vi "Query Multi Eval Meas List Power Spectral Density Limit Check Results.vi"(8 "error in (no error)":errorcluster, 9 "Result Type (Current)":i32(ring) items=["Current"=0, "Average"=1, "Maximum"=4, "Minimum"=5], 10 "Instance (1)":T1=1, 11 "VISA resource name":refnum<visa-resource-name>) -> (0 "error out":errorcluster, 1 "Limit Check Results":i32[](array[numeric]), 2 "Reliability":i32, 3 "VISA resource name out":refnum<visa-resource-name>)   [LabVIEW 2020, in "Rohde&Schwarz CMWXP NR FR1 Measurement.lvlib"]
doc: "Return RB power limit check results (power spectral density) for all measured list mode segments.\n\nAttributes:\nRSCMWXPNRFR1M_ATTR_QUERY_MULTI_EVAL_MEAS_LIST_POWER_SPECTRAL_DENSITY_CURRENT_LIMIT_CHECK_RESULTS\nRSCMWXPNRFR1M_ATTR_QUERY_MULTI_EVAL_MEAS_LIST_POWER_SPECTRAL_DENSITY_AVERAGE_LIMIT_CHECK_RESULTS\nRSCMWXPNRFR1M_ATTR_QUERY_MULTI_EVAL_MEAS_LIST_POWER_SPECTRAL_DENSITY_MAXIMUM_LIMIT_CHECK_RESULTS\nRSCMWXPNRFR1M_ATTR_QUERY_MULTI_EVAL_MEAS_LIST_POWER_SPECTRAL_DENSITY_MINIMUM_LIMIT_CHECK_RESULTS\n\nRemote-control commands:\nCALCulate:NRSub:MEAS<i>:MEValuation:LIST:MODulation:PSD:CURRent?\nCALCulate:NRSub:MEAS<i>:MEValuation:LIST:MODulation:PSD:AVERage?\nCALCulate:NRSub:MEAS<i>:MEValuation:LIST:MODulation:PSD:MAXimum?\nCALCulate:NRSub:MEAS<i>:MEValuation:LIST:MODulation:PSD:MINimum?"
uses:
  <instrlib>/Rohde&Schwarz CMWXP NR FR1 Measurement/Rohde&Schwarz CMWXP NR FR1 Measurement.lvlib
  <instrlib>/Rohde&Schwarz CMWXP NR FR1 Measurement/Private/_Instance.ctl
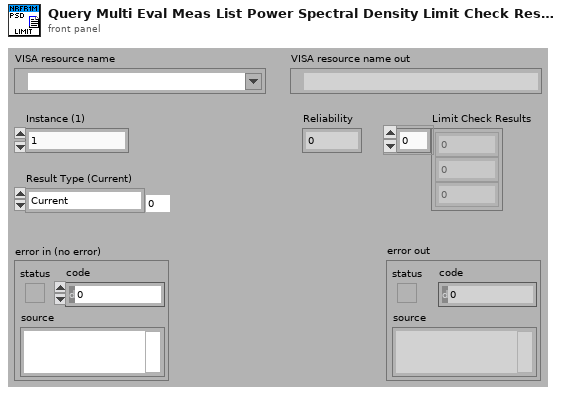
[diagram p1: front panel]
types:
  T1 = typedef "Rohde&Schwarz CMWXP NR FR1 Measurement.lvlib/_Instance.ctl" = i32
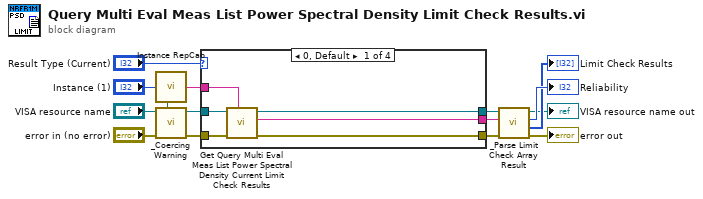
[diagram p0: block diagram]
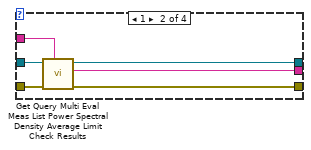
[diagram p2: hidden frame]
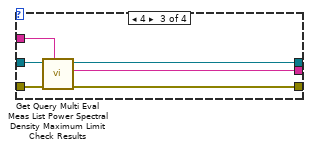
[diagram p3: hidden frame]
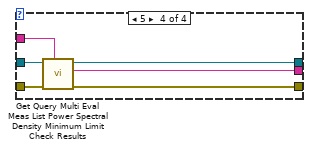
[diagram p4: hidden frame]
diagram:
  n1 = call <instrlib>:"Instance RepCap.vi"("Instance In"="Instance (1)") -> ("In Range?"=w13:bool, "RepCap Identifier Out"=w9:string)  [unwired: 1 in]
  n2 = call <instrlib>:"_Coercing Warning.vi"("In Range?"=w13, "error in (no error)"="error in (no error)", "VISA resource name"="VISA resource name") -> ("error out"=w10:errorcluster, "VISA resource name out"=w11:refnum<visa-resource-name>)  [unwired: 7 in]
  n3 = case shown="0, Default" "Result Type (Current)" {
    tunnel: w11 -> [w21 w27 w33 w39]
    tunnel: w10 -> [w20 w26 w32 w38]
    tunnel: w9 -> [w19 w25 w31 w37]
    tunnel: [w18 w24 w30 w36] -> w5
    tunnel: [w17 w23 w29 w35] -> w6
    tunnel: [w16 w22 w28 w34] -> w7
    frame 0, Default {
      n4 = call "Get Query Multi Eval Meas List Power Spectral Density Current Limit Check Results"("Repeated Capabilities"=w19, "error in (no error)"=w20, "instrument handle"=w21) -> ("error out"=w16:errorcluster, "Query Multi Eval Meas List Power Spectral Density Current Limit Check Results"=w17:string, "instrument handle out"=w18:refnum<visa-resource-name>)  [unwired: 6 in]
    }
    frame 1 {
      n5 = call "Get Query Multi Eval Meas List Power Spectral Density Average Limit Check Results"("Repeated Capabilities"=w25, "error in (no error)"=w26, "instrument handle"=w27) -> ("error out"=w22:errorcluster, "Query Multi Eval Meas List Power Spectral Density Average Limit Check Results"=w23:string, "instrument handle out"=w24:refnum<visa-resource-name>)  [unwired: 6 in]
    }
    frame 4 {
      n6 = call "Get Query Multi Eval Meas List Power Spectral Density Maximum Limit Check Results"("Repeated Capabilities"=w31, "error in (no error)"=w32, "instrument handle"=w33) -> ("error out"=w28:errorcluster, "Query Multi Eval Meas List Power Spectral Density Maximum Limit Check Results"=w29:string, "instrument handle out"=w30:refnum<visa-resource-name>)  [unwired: 6 in]
    }
    frame 5 {
      n7 = call "Get Query Multi Eval Meas List Power Spectral Density Minimum Limit Check Results"("Repeated Capabilities"=w37, "error in (no error)"=w38, "instrument handle"=w39) -> ("error out"=w34:errorcluster, "Query Multi Eval Meas List Power Spectral Density Minimum Limit Check Results"=w35:string, "instrument handle out"=w36:refnum<visa-resource-name>)  [unwired: 6 in]
    }
  }
  n8 = call <instrlib>:"_Parse Limit Check Array Result.vi"("error in (no error)"=w7, "Input String"=w6, "VISA resource name"=w5) -> ("error out"=→"error out":errorcluster, "Results"=→"Limit Check Results":i32[], "Reliability"=→"Reliability":i32, "VISA resource name out"=→"VISA resource name out":refnum<visa-resource-name>)  [unwired: 3 in, 1 out]
